vi "TestDocu.vi"() -> ()   [LabVIEW 2022 SP3]
panel:
  out "Time has Elapsed 2":bool caption="Time has Elapsed"
  out "Elapsed Time (s)":dbl
  out "Time has Elapsed":bool
  in  "Boolean":bool
  in  "stop":bool
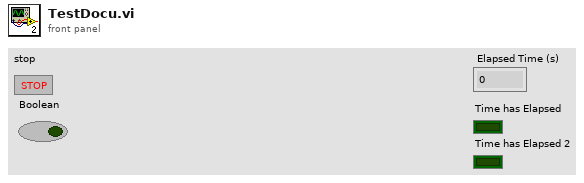
[diagram p1: front panel]
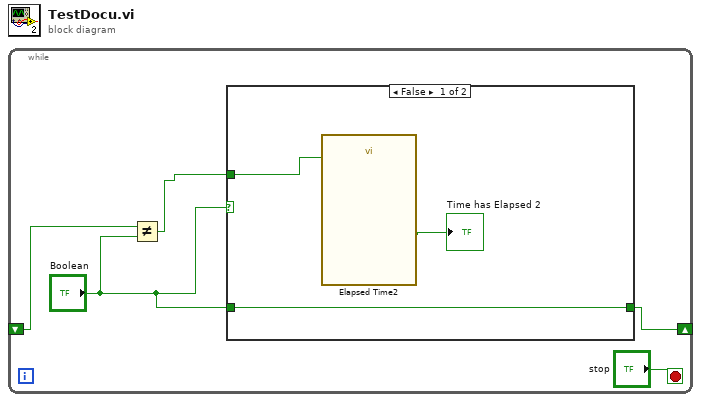
[diagram p0: block diagram]
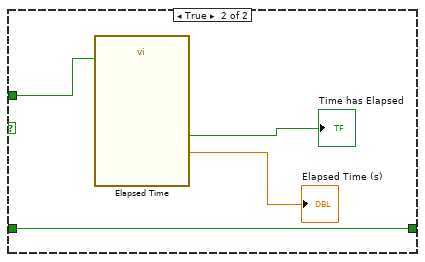
[diagram p2: hidden frame]
diagram:
  n1 = while {
    shift-right: [w2] -> _
    shift-left: _ -> [w4]
    stop <- "stop" stop-if-true
    n2 = Not Equal?(x=w4, y="Boolean") -> (x != y?=w1:bool)
    n3 = case shown="False" "Boolean" {
      tunnel: "Boolean" -> [w8 w11]
      tunnel: [w8 w11] -> w2
      tunnel: w1 -> [w7 w9]
      frame False {
        n4 = call "Elapsed Time2"("Reset"=w7) -> ("Time has Elapsed"=→"Time has Elapsed 2":bool)  [unwired: 11 in, 7 out]
      }
      frame True {
        n5 = call "Elapsed Time"("Reset"=w9) -> ("Elapsed Time (s)"=→"Elapsed Time (s)":dbl, "Time has Elapsed"=→"Time has Elapsed":bool)  [unwired: 11 in, 6 out]
      }
    }
  }
